vi "UpdateGeometricParameters.vi"(8 "error in":errorcluster, 9 "Shoulder Joint Center":dbl[](array[numeric]), 10 "Arm Lengths":dbl[](array[numeric]), 11 "Exoskeleon in":refnum<class "Exoskeleon.lvclass">) -> (0 "error out":errorcluster, 3 "Exoskeleon out":refnum<class "Exoskeleon.lvclass">)   [LabVIEW 2014, in "Exoskeleon.lvclass"]
uses:
  Classes/CAREX_Classes_old/Exoskeleton/Exoskeleon.lvclass
  Classes/CAREX_Classes_old/Exoskeleton/Exoskeleton_SetArmLengths.vi
  Classes/CAREX_Classes_old/Exoskeleton/Exoskeleton_SetShoulderCuffOffset.vi
  Classes/CAREX_Classes_old/Exoskeleton/Exoskeleton_SetLinkCOMs.vi
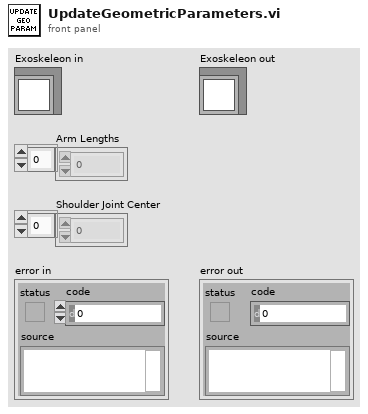
[diagram p1: front panel]
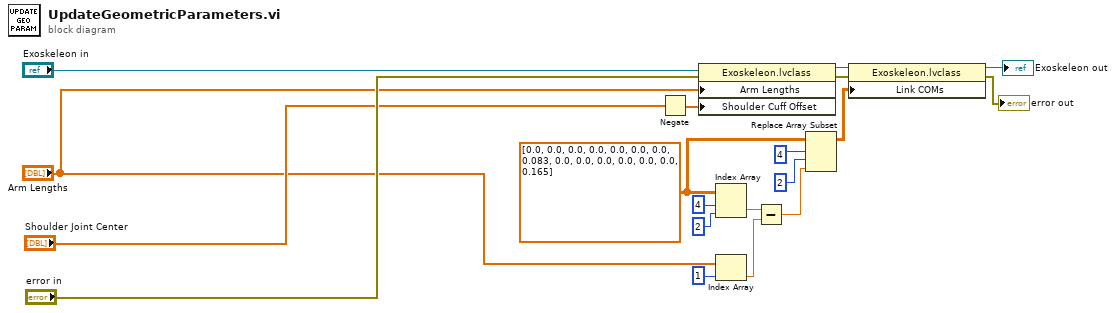
[diagram p0: block diagram]
diagram:
  w2 = dbl[][] [[0.0, 0.0, 0.0], [0.0, 0.0, 0.0], [0.0, 0.083, 0.0], [0.0, 0.0, 0.0], [0.0, 0.0, 0.165]]
  n1 = Negate(x="Shoulder Joint Center") -> (-x=w1:dbl[])
  n2 = property class="Exoskeleon.lvclass"(reference="Exoskeleon in", error in="error in", "Arm Lengths"="Arm Lengths", "Shoulder Cuff Offset"=w1) -> (reference out=w4:refnum<class "Exoskeleon.lvclass">, error out=w17:errorcluster)
  n3 = Index Array(array=w2, index (row)=4, index (col)=2 ("index (row)")) -> (element=w9:dbl)
  n4 = Index Array(array="Arm Lengths", index=1) -> (element=w10:dbl)
  n5 = Subtract(x=w9, y=w10) -> (x-y=w13:dbl)
  n6 = Replace Array Subset(array=w2, new element=w13, index (row)=4, index (col)=2 ("index (row)")) -> (w14:dbl[][])
  n7 = property class="Exoskeleon.lvclass"(reference=w4, error in=w17, "Link COMs"=w14) -> (reference out=→"Exoskeleon out":refnum<class "Exoskeleon.lvclass">, error out=→"error out":errorcluster)
